vi "cc_read.vi"(3 "error in (no error)":errorcluster, 5 "VISA In":refnum<visa-resource-name>) -> (0 "error out":errorcluster, 1 "Input String":string, 2 "VISA Out":refnum<visa-resource-name>)   [LabVIEW 2020]
doc: "Read a string from Cryocon"
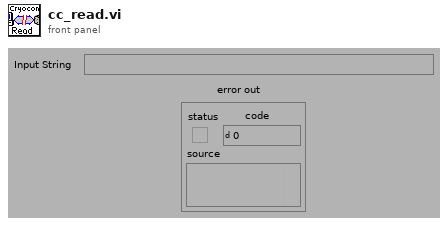
[diagram p1: front panel]
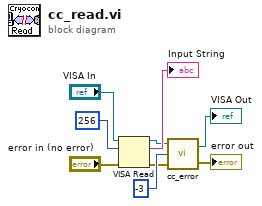
[diagram p0: block diagram]
diagram:
  n1 = VISA Read(VISA resource name="VISA In", byte count=u32 256, error in (no error)="error in (no error)") -> (VISA resource name out=w4:refnum<visa-resource-name>, read buffer=→"Input String":string, error out=w3:errorcluster)  [unwired: 1 out]
  n2 = call "cc_error.vi"("error in (no error)"=w3, "Error code"=-3, "VISA In"=w4) -> ("error out"=→"error out":errorcluster, "VISA out"=→"VISA Out":refnum<visa-resource-name>)
